vi "SingleActionEngineSANDBOX.vi"() -> ()   [LabVIEW 2022 SP3]
uses:
  ActionEngineEnum.ctl
  C:/Users/mnopl/OneDrive/Documents/PhiThetaScanning/Thorlabs.MotionControl.Controls.dll
  Thorlabs.MotionControl.Controls.dll
panel:
  in  "Settings":T1={"Step Size (mm)"=10.0, "Initial Position"=0.0, "Move Absolute/Relative Position"=0.0, "Step Delay (ms)"=0, "Velocity (mm/s)"=1.5, "Acceleration (mm/s^2)"=1.0} {"Step Size (mm)" min=0.00046 format="%.8f"}
  in  "SerialNumber":string="26004239"
  in  "KCubeStepperControl":refnum<k24>(container)
  out "Current Position (mm)":dbl
  out "error out":errorcluster
  in  "stop":bool
  in  "Action":T2=enum."Done"
  # "INPUT"
  # "OUTPUT"
  # "\"DONE\" is the default state; it will not execute when you press \"RUN\". The first state executes when you first change the state,\ni.e. if it is initially \"DONE\", nothing will happen until you change it to \"Open Connection\"."
  # "\"MOVE ABSOLUTE\" homes motor before moving to \n\"MOVE POSITION\", regardless of step size."
  # "\"SETTINGS\" Controls velocity and acceleration, must be updated values before calling."
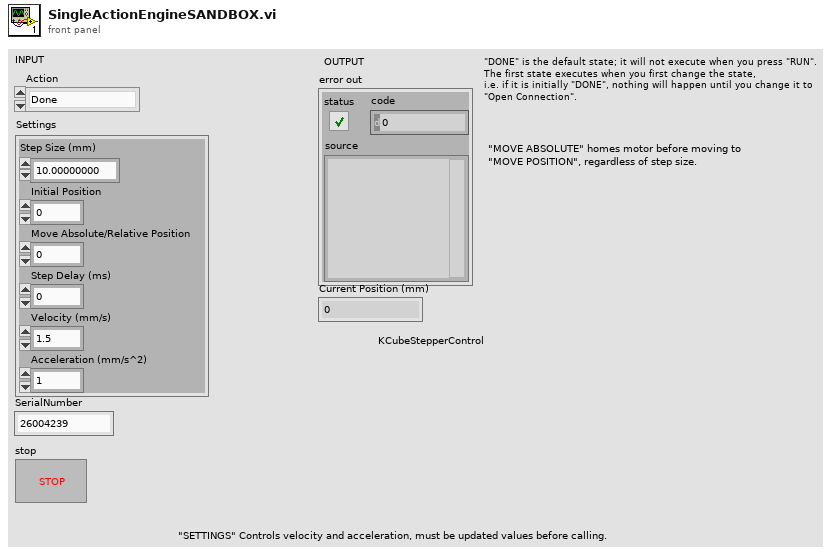
[diagram p1: front panel]
types:
  T1 = cluster{"Step Size (mm)":sgl, "Initial Position":dbl, "Move Absolute/Relative Position":dbl, "Step Delay (ms)":u32, "Velocity (mm/s)":dbl, "Acceleration (mm/s^2)":dbl}
  T2 = typedef "ActionEngineEnum.ctl" = enum16{"Open Connection", "Done", "Get Position", "Settings", "Home", "Move Absolute", "Move Relative", "Step", "Stop Action", "Close Connection"}
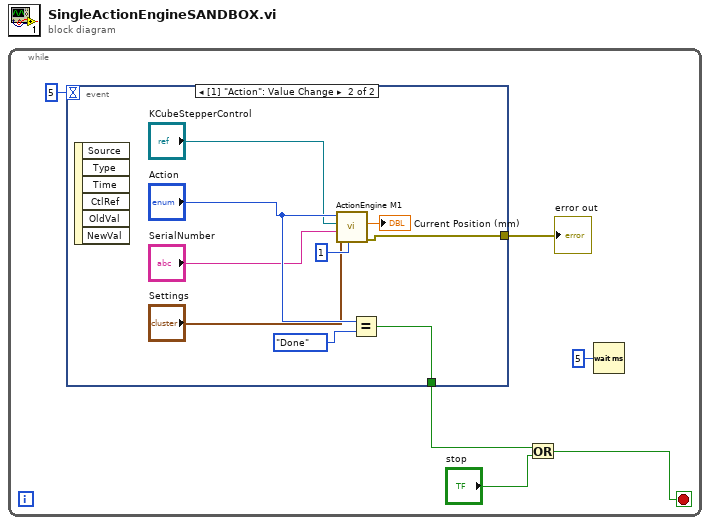
[diagram p0: block diagram]
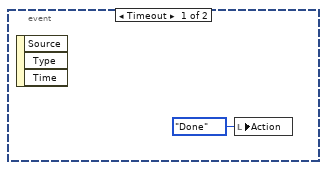
[diagram p2: hidden frame]
diagram:
  n1 = while {
    stop <- w1 stop-if-true
    n2 = event shown="[1] \"Action\": Value Change" {
      selector: _ -> [_ _]
      dyn-events: _ -> [_ _]
      timeout: 5 -> [_ _]
      tunnel: [_ w16] -> w4
      tunnel: [_ w13] -> w3
      event Timeout {
        n3 = event-data() -> ()  [unwired: 1 in, 3 out]
        n4 = local write "Action"(ActionEngineEnum."Done" ("Action")) -> ()
      }
      event Value Change {
        n5 = event-data() -> ()  [unwired: 1 in, 6 out]
        n6 = call "ActionEngine M1.vi"("ChannelNumber"=1, "Settings"="Settings", "SerialNumber"="SerialNumber", "KCubeStepperControl"="KCubeStepperControl", "Action"="Action") -> ("error out"=w16:errorcluster, "Current Position"=→"Current Position (mm)":dbl)  [unwired: 4 in]
        n7 = Equal?(x="Action", y=ActionEngineEnum."Done" ("Action")) -> (x = y?=w13:bool)
      }
    }
    "error out" <- w4
    n8 = Or(x=w3, y="stop") -> (x .or. y?=w1:bool)
    n9 = Wait (ms)(milliseconds to wait=u32 5) -> ()  [unwired: 1 out]
  }
